vi "Send_DET_CLIENT_READ.vi"(8 "error in (no error)":errorcluster, 9 "error to send":errorcluster, 10 "Signals so Send":T1, 11 "Queue in":refnum<queue>) -> (0 "error out":errorcluster)   [LabVIEW 2020, in "Detector.lvclass"]
uses:
  Detector.lvclass
  dependecies/ControlsVIs/Clusters-def/Det-Reply-to-Read.ctl
  dependecies/ControlsVIs/Clusters-def/Def_signals_from_DET.ctl
  dependecies/ControlsVIs/Clusters-def/Standard Command.ctl
  dependecies/ControlsVIs/Clusters-def/SERVER-Commands.ctl
  Control/Control-Server/Control-Server.lvclass
panel:
  in  "?":T2
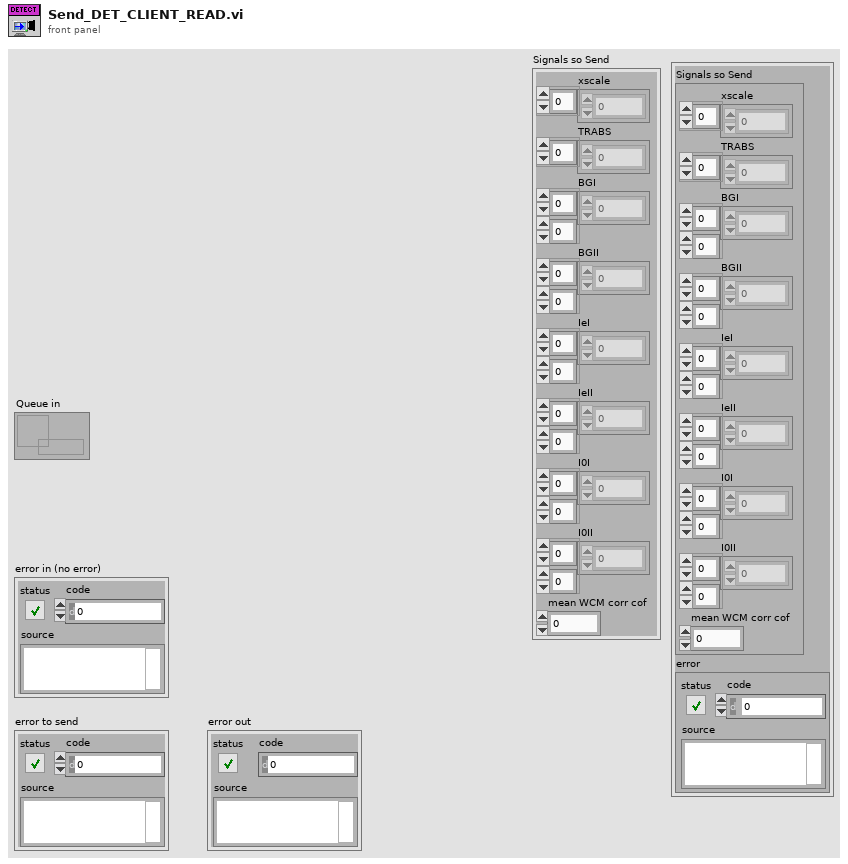
[diagram p1: front panel]
types:
  T1 = typedef "Detector.lvclass/Def_signals_from_DET.ctl" = cluster{"xscale":sgl[], "TRABS":sgl[], "BGI":sgl[][], "BGII":sgl[][], "IeI":sgl[][], "IeII":sgl[][], "I0I":sgl[][], "I0II":sgl[][], "mean WCM corr cof":dbl}
  T2 = typedef "Detector.lvclass/Det-Reply-to-Read.ctl" = cluster{"Signals so Send":T1, "error":errorcluster}
  T3 = typedef "Control-Server.lvclass/SERVER-Commands.ctl" = string
  T4 = typedef "Standard Command.ctl" = cluster{"command":string, "data":variant}
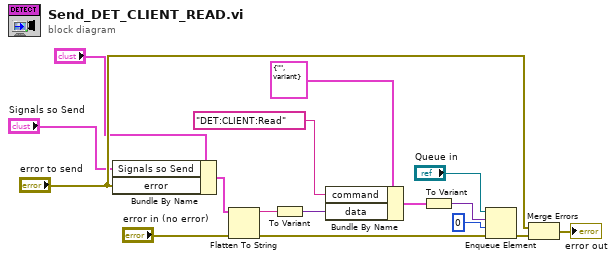
[diagram p0: block diagram]
diagram:
  n1 = Bundle By Name(cluster="?", "Signals so Send"="Signals so Send", "error"="error to send") -> (w7:T2)
  n2 = Flatten To String(anything=w7, error in (no error)="error in (no error)") -> (data string=w8:string, error out=w13:errorcluster)  [unwired: 2 in, 1 out]
  n3 = To Variant(anything=w8) -> (Variant=w5:variant)
  n4 = Bundle By Name(cluster=T4 {"command"="", "data"=variant} ("input cluster"), "command"=T3 "DET:CLIENT:Read" ("Commands"), "data"=w5) -> (w9:T4)
  n5 = To Variant(anything=w9) -> (Variant=w10:variant)
  n6 = Enqueue Element(queue="Queue in", element=w10, timeout in ms (-1)=0 ("timeout en ms (-1)"), error in (no error)=w13) -> (error out=w14:errorcluster)  [unwired: 2 out]
  n7 = Merge Errors("error to send", w14) -> (→"error out":errorcluster)
